vi "Configure Post Operating Point Measurements.vi"(8 "error in (no error)":errorcluster, 11 "QPA Measurement in":refnum<class "QPA Measurement.lvclass">) -> (0 "error out":errorcluster, 3 "QPA Measurement out":refnum<class "QPA Measurement.lvclass">)   [LabVIEW 2016, in "QPA Measurement.lvlib" / "QPA Measurement.lvclass"]
uses:
  QPA Measurement.lvclass
  C:/Projects/STS/Common/Sequence Automation/Plugins/Measurement Interface.lvlibp/Measurement Interface.lvclass
  C:/Projects/STS/Common/Sequence Automation/Plugins/FPF.lvlibp/Factory Plugin Framework.lvclass
  QPA Measurement.lvclass/QPA Measurement.ctl
  Plugins/Measurement Interface.lvlibp/Private Methods/Measurement Parameters/Read Measurement Parameters.vi
  Plugins/Measurement Interface.lvlibp/Private Methods/Measurement Parameters/Write Measurement Parameters.vi
  Plugins/String Database.lvlibp/String Database.lvclass
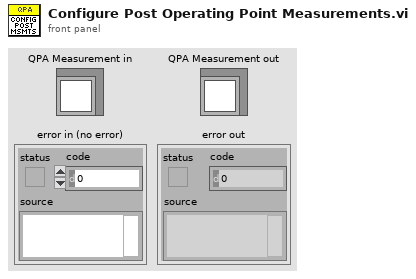
[diagram p1: front panel]
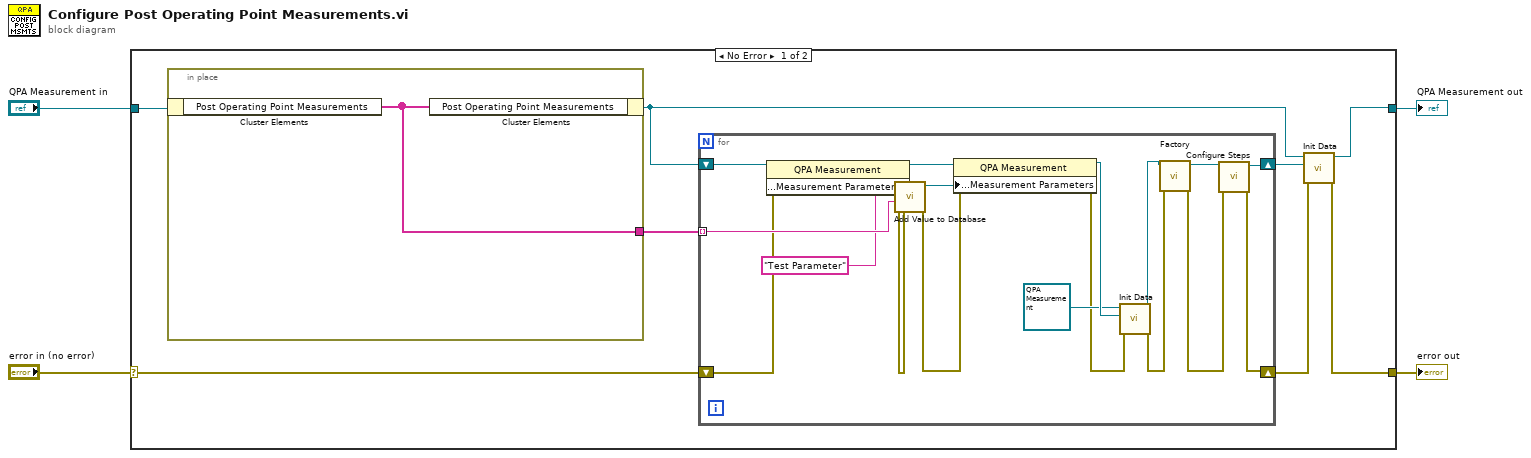
[diagram p0: block diagram]
diagram:
  n1 = case shown="No Error" "error in (no error)" {
    selector: "error in (no error)" -> [w10 w33]
    tunnel: [w6 w33] -> w3
    tunnel: [w7 w32] -> w1
    tunnel: "QPA Measurement in" -> [w12 w32]
    frame No Error {
      n2 = in-place {
        in-place-border: [w31] -> w11
        n3 = in-place-cluster #1(w12) -> ("Post Operating Point Measurements"=w31:string[])
        n4 = in-place-cluster #1("Post Operating Point Measurements"=w31) -> (w8:refnum<class "QPA Measurement.lvclass">)
      }
      n5 = for {
        tunnel: w11 -> [w28] mode=indexing
        shift-right: [w19] -> w5
        shift-left: w10 -> [w27]
        shift-right: [w18] -> w9
        shift-left: w8 -> [w30]
        n6 = property class="QPA Measurement"(reference=w30, error in=w27) -> (reference out=w25:refnum<class "QPA Measurement.lvclass">, error out=w26:errorcluster, "Protected Methods:Measurement Parameters"=w29:refnum<class "String Database.lvclass">)
        n7 = call "Add Value to Database.vi"("error in (no error)"=w26, "Entry Value"=w28, "Entry Name"="Test Parameter", "Dictionary In"=w29) -> ("error out"=w23:errorcluster, "Dictionary Out"=w24:refnum<class "String Database.lvclass">)  [unwired: 5 in, 1 out]
        n8 = property class="QPA Measurement"(reference=w25, error in=w23, "Protected Methods:Measurement Parameters"=w24) -> (reference out=w16:refnum<class "QPA Measurement.lvclass">, error out=w14:errorcluster)
        n9 = call-dynamic "Init Data.vi"("error in (no error)"=w14, "Data Object"=w16, "QPA Measurement in"=refnum<class "QPA Measurement.lvclass"> refnum) -> ("error out"=w13:errorcluster, "QPA Measurement out"=w17:refnum<class "QPA Measurement.lvclass">)  [unwired: 7 in]
        n10 = call-dynamic "Factory.vi"("error in (no error)"=w13, "QPA Measurement in"=w17) -> ("error out"=w20:errorcluster, "QPA Measurement out"=w21:refnum<class "QPA Measurement.lvclass">)  [unwired: 8 in]
        n11 = call-dynamic "Configure Steps.vi"("error in (no error)"=w20, "QPA Measurement in"=w21) -> ("error out"=w19:errorcluster, "QPA Measurement out"=w18:refnum<class "QPA Measurement.lvclass">)  [unwired: 8 in]
      }
      n12 = call-dynamic "Init Data.vi"("error in (no error)"=w5, "Data Object"=w9, "QPA Measurement in"=w8) -> ("error out"=w6:errorcluster, "QPA Measurement out"=w7:refnum<class "QPA Measurement.lvclass">)  [unwired: 7 in]
    }
    frame Error {
    }
  }
  "error out" <- w3
  "QPA Measurement out" <- w1
